vi "TC560-Read Data.vi"(8 "error in":errorcluster, 11 "VISA Resource Name In":refnum<visa-resource-name>) -> (0 "error out":errorcluster, 1 "Voltage":dbl, 2 "Resistance":dbl, 3 "VISA Resource Name Out":refnum<visa-resource-name>)   [LabVIEW 2018]
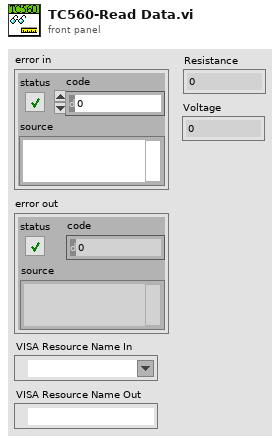
[diagram p1: front panel]
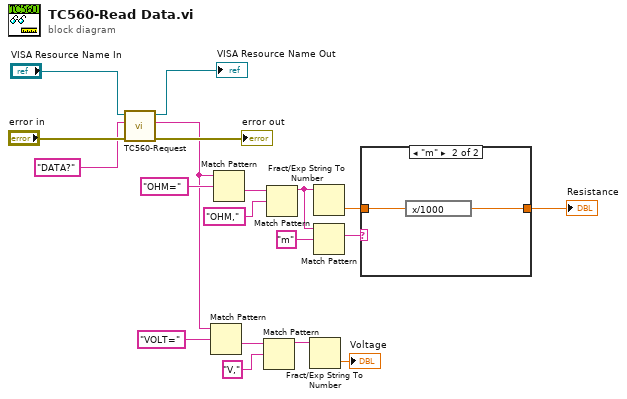
[diagram p0: block diagram]
diagram:
  n1 = call "TC560-Request.vi"("error in"="error in", "Command"="DATA?" ("string"), "VISA Resource Name In"="VISA Resource Name In") -> ("error out"=→"error out":errorcluster, "Respond"=w8:string, "VISA Resource Name Out"=→"VISA Resource Name Out":refnum<visa-resource-name>)  [unwired: 6 in]
  n2 = Match Pattern(string=w8, regular expression="VOLT=") -> (after substring=w11:string)  [unwired: 1 in, 3 out]
  n3 = Match Pattern(string=w8, regular expression="OHM=") -> (after substring=w14:string)  [unwired: 1 in, 3 out]
  n4 = Match Pattern(string=w11, regular expression="V,") -> (before substring=w13:string)  [unwired: 1 in, 3 out]
  n5 = Match Pattern(string=w14, regular expression="OHM,") -> (before substring=w5:string)  [unwired: 1 in, 3 out]
  n6 = Fract/Exp String To Number(string=w13) -> (number=→"Voltage":dbl)  [unwired: 3 in, 1 out]
  n7 = Fract/Exp String To Number(string=w5) -> (number=w4:dbl)  [unwired: 3 in, 1 out]
  n8 = Match Pattern(string=w5, regular expression="m") -> (match substring=w1:string)  [unwired: 1 in, 3 out]
  n9 = case shown="\"m\"" w1 {
    tunnel: w4 -> [w20 w22]
    tunnel: [w20 w21] -> w3
    frame "False", Default {
    }
    frame "m" {
      n10 = expression code="x/1000"(w22) -> (w21:dbl)
    }
  }
  "Resistance" <- w3
